vi "TranslatorBooster Scan DataType.vi"(11 "whole match":string) -> (1 "usnigned?":bool, 2 "ref?":bool, 3 "pointer?":bool, 4 "dataType":string, 5 "type":string)   [LabVIEW 2014, in "Complex Numbers.lvlib"]
uses:
  <vilib>/Aledyne-TSXperts/Arduino Compatible Compiler for LabVIEW/addons/Complex Numbers/Complex Numbers.lvlib
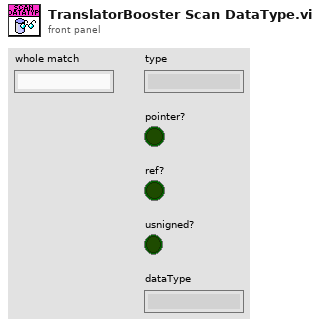
[diagram p1: front panel]
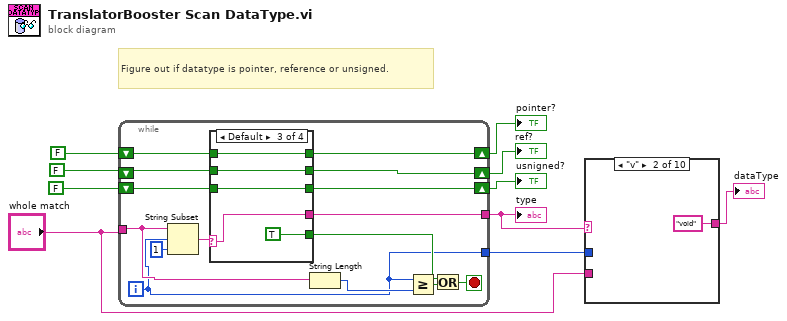
[diagram p0: block diagram]
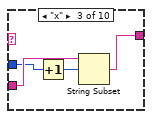
[diagram p3: hidden frame]
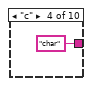
[diagram p4: hidden frame]
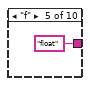
[diagram p5: hidden frame]
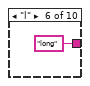
[diagram p6: hidden frame]
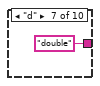
[diagram p7: hidden frame]
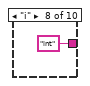
[diagram p8: hidden frame]
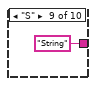
[diagram p9: hidden frame]
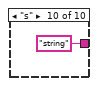
[diagram p10: hidden frame]
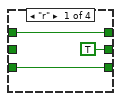
[diagram p11: hidden frame]
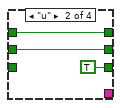
[diagram p12: hidden frame]
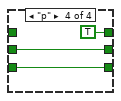
[diagram p13: hidden frame]
diagram:
  # "Figure out if datatype is pointer, reference or unsigned."
  n1 = while {
    tunnel: "whole match" -> [w17]
    shift-right: [w22] -> w4
    shift-left: FALSE -> [w23]
    shift-right: [w21] -> w5
    shift-left: FALSE -> [w20]
    shift-right: [w18] -> w6
    shift-left: FALSE -> [w19]
    tunnel: [w14] -> w7
    tunnel: [w11] -> w9
    i -> [w11]
    stop <- w15 stop-if-true
    n2 = String Subset(string=w17, offset (0)=w11, length (rest)=1 ("length (rest)")) -> (substring=w24:string)
    n3 = case shown="Default" w24 {
      selector: w24 -> [_ _ w33 _]
      tunnel: w23 -> [w27 w29 w36 _]
      tunnel: [w27 w29 w36 TRUE] -> w22
      tunnel: [TRUE w30 w35 w38] -> w21
      tunnel: w20 -> [_ w30 w35 w38]
      tunnel: w19 -> [w26 _ w34 w37]
      tunnel: [w26 TRUE w34 w37] -> w18
      tunnel: [_ _ w33 _] -> w14
      tunnel: [_ _ TRUE _] -> w13
      frame "r" {
      }
      frame "u" {
      }
      frame Default {
      }
      frame "p" {
      }
    }
    n4 = String Length(string=w17) -> (length=w12:i32)
    n5 = Greater Or Equal?(x=w11, y=w12) -> (x >= y?=w16:bool)
    n6 = Or(x=w13, y=w16) -> (x .or. y?=w15:bool)
  }
  "pointer?" <- w4
  "ref?" <- w5
  "usnigned?" <- w6
  "type" <- w7
  n7 = case shown="\"v\"" w7 {
    tunnel: "whole match" -> [_ _ w44 _ _ _ _ _ _ _]
    tunnel: w9 -> [_ _ w43 _ _ _ _ _ _ _]
    tunnel: [_ "void" ("whole match") w42 "char" ("whole match") "float" ("whole match") "long" ("whole match") "double" ("whole match") "int" ("whole match") "String" ("whole match") "string" ("whole match")] -> w10
    frame Default {
    }
    frame "v" {
    }
    frame "x" {
      n8 = Increment(x=w43) -> (x+1=w41:i32)
      n9 = String Subset(string=w44, offset (0)=w41) -> (substring=w42:string)  [unwired: 1 in]
    }
    frame "c" {
    }
    frame "f" {
    }
    frame "l" {
    }
    frame "d" {
    }
    frame "i" {
    }
    frame "S" {
    }
    frame "s" {
    }
  }
  "dataType" <- w10
